vi "Set Wire Label.vi"(8 "error in (no error)":errorcluster, 9 "QD Combo Box Ref":refnum<vi>, 10 "Shift Not Pressed?":bool, 11 "Wire in":refnum<vi>) -> (0 "error out":errorcluster)   [LabVIEW 2017]
uses:
  <vilib>/Utility/miscctls.llb/LVPointTypeDef.ctl
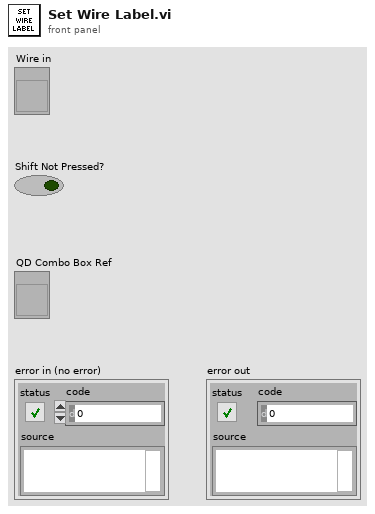
[diagram p1: front panel]
types:
  T1 = typedef "LVPointTypeDef.ctl" = cluster{"Horizontal":i16, "Vertical":i16}
  T2 = cluster{"Position":cluster{"h":i16, "v":i16}, "Flags":i32, "Type":enum32{"LooseEnd", "Endpoint", "Bend", "Junction"}, "Up Joint Index":i16, "Down Joint Index":i16, "Left Joint Index":i16, "Right Joint Index":i16}[]
  T3 = typedef "LVBoundsTypeDef.ctl" = cluster{"Width":u32, "Height":u32}
  T4 = cluster{"Position":cluster{"h":i16, "v":i16}, "Flags":i32, "Type":enum32{"LooseEnd", "Endpoint", "Bend", "Junction"}, "Up Joint Index":i16, "Down Joint Index":i16, "Left Joint Index":i16, "Right Joint Index":i16}
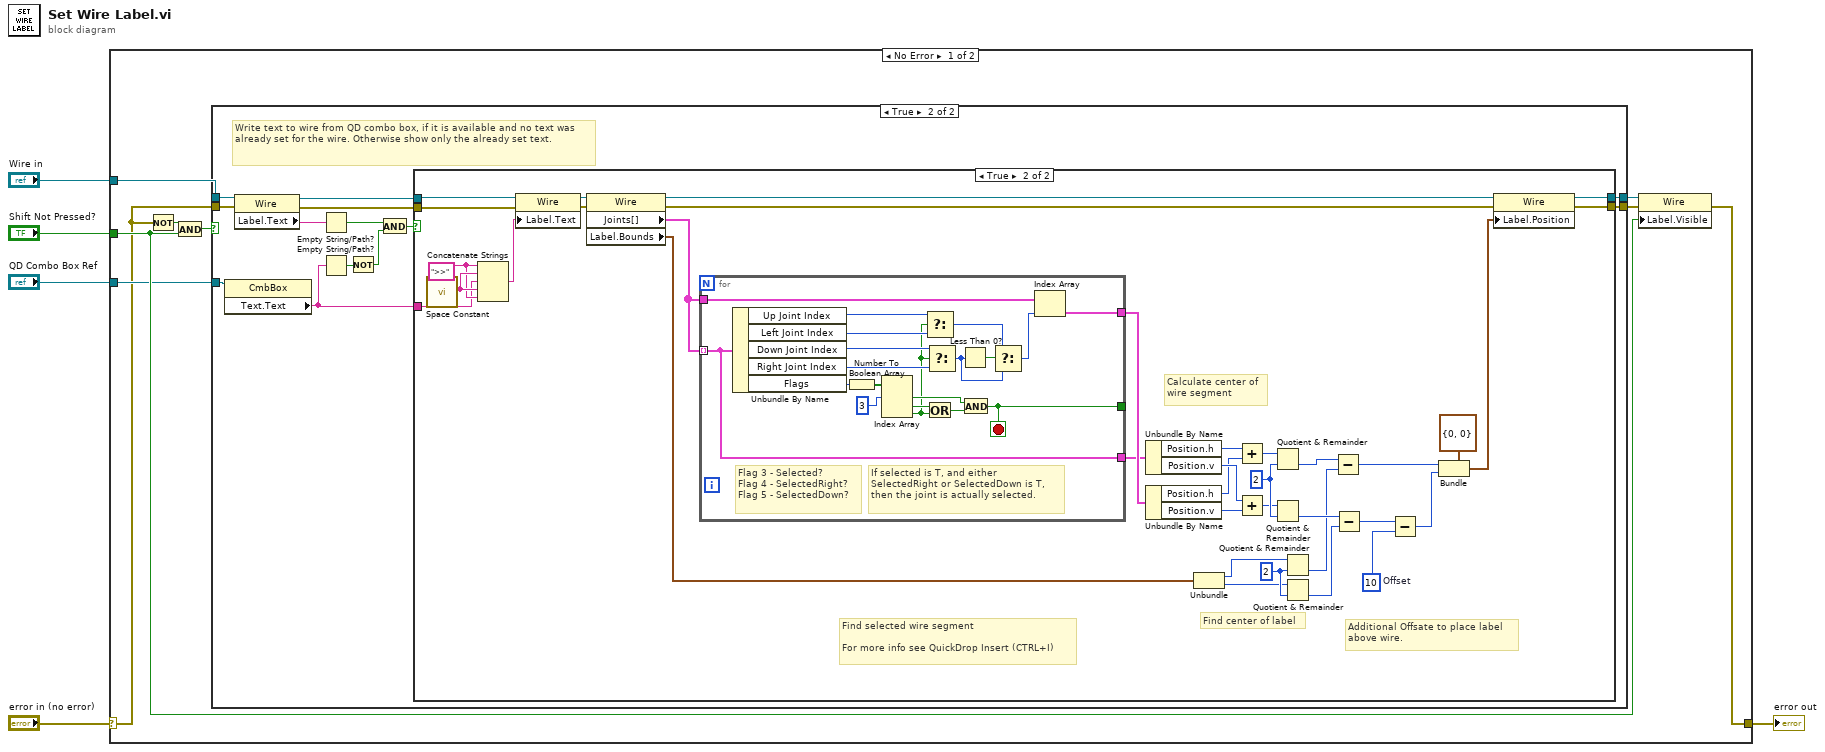
[diagram p0: block diagram]
diagram:
  n1 = case shown="No Error" "error in (no error)" {
    selector: "error in (no error)" -> [w12 w87]
    tunnel: [w6 w87] -> w5
    tunnel: "Shift Not Pressed?" -> [w14 _]
    tunnel: "QD Combo Box Ref" -> [w13 _]
    tunnel: "Wire in" -> [w7 _]
    frame No Error {
      n2 = Not(x=w12) -> (.not. x?=w11:bool)
      n3 = And(x=w11, y=w14) -> (x .and. y?=w10:bool)
      n4 = case shown="True" w10 {
        tunnel: w13 -> [_ w29]
        tunnel: w7 -> [w16 w26]
        tunnel: [w16 w28] -> w8
        tunnel: [w15 w27] -> w9
        tunnel: w12 -> [w15 w25]
        frame False {
        }
        frame True {
          # "Write text to wire from QD combo box, if it is available and no text was already set for the wire. Otherwise show only the already set text."
          n5 = property class="CmbBox"(reference=w29) -> ("Text.Text"=w21:string)  [unwired: 1 in, 2 out]
          n6 = property class="Wire"(reference=w26, error in=w25) -> (reference out=w23:refnum<vi>, error out=w24:errorcluster, "Label.Text"=w22:string)
          n7 = Empty String/Path?(string/path=w22) -> (empty?=w17:bool)
          n8 = Empty String/Path?(string/path=w21) -> (empty?=w20:bool)
          n9 = Not(x=w20) -> (.not. x?=w18:bool)
          n10 = And(x=w17, y=w18) -> (x .and. y?=w19:bool)
          n11 = case shown="True" w19 {
            tunnel: [w31 w48] -> w28
            tunnel: [w30 w47] -> w27
            tunnel: w24 -> [w30 w64]
            tunnel: w23 -> [w31 w63]
            tunnel: w21 -> [_ w62]
            frame False {
            }
            frame True {
              w36 = u32 10  # Offset
              w43 = i16 2 ("y")
              w56 = i16 2 ("y")
              w66 = ">>"
              # "Calculate center of\nwire segment"
              # "Find center of label"
              # "Additional Offsate to place label\nabove wire."
              # "Find selected wire segment\n\nFor more info see QuickDrop Insert (CTRL+I)"
              n12 = call <vilib>:"Space Constant.vi"() -> ("String"=w67:string)
              n13 = Concatenate Strings(w66, w67, w62, w67, w66) -> (w61:string)
              n14 = property class="Wire"(reference=w63, error in=w64, "Label.Text"=w61) -> (reference out=w65:refnum<vi>, error out=w59:errorcluster)
              n15 = property class="Wire"(reference=w65, error in=w59) -> (reference out=w60:refnum<vi>, error out=w46:errorcluster, "Joints[]"=w49:T2, "Label.Bounds"=w44:T3)
              n16 = for {
                tunnel: w49 -> [w80] mode=indexing
                tunnel: w49 -> [w79]
                tunnel: [w80] -> w51
                tunnel: [w78] -> w52
                tunnel: [w68] -> _
                stop <- w68 stop-if-true
                # "If selected is T, and either SelectedRight or SelectedDown is T, then the joint is actually selected."
                # "Flag 3 - Selected?\nFlag 4 - SelectedRight?\nFlag 5 - SelectedDown?"
                n17 = Unbundle By Name(w80) -> ("Up Joint Index"=w75:i16, "Left Joint Index"=w74:i16, "Down Joint Index"=w77:i16, "Right Joint Index"=w76:i16, "Flags"=w86:i32)
                n18 = Number To Boolean Array(number=w86) -> (Boolean array=w85:bool[])
                n19 = Index Array(array=w85, index #1=3 ("index")) -> (element #1=w81:bool, element #2=w82:bool, element #3=w73:bool)  [unwired: 2 in]
                n20 = Select(t=w75, s=w73, f=w74) -> (s? t:f=w70:i16)
                n21 = Or(x=w82, y=w73) -> (x .or. y?=w83:bool)
                n22 = Select(t=w77, s=w73, f=w76) -> (s? t:f=w69:i16)
                n23 = Less Than 0?(x=w69) -> (x < 0?=w71:bool)
                n24 = And(x=w81, y=w83) -> (x .and. y?=w68:bool)
                n25 = Select(t=w70, s=w71, f=w69) -> (s? t:f=w72:i16)
                n26 = Index Array(array=w79, index=w72) -> (element=w78:T4)
              }
              n27 = Unbundle By Name(w51) -> ("Position.h"=w35:i16, "Position.v"=w58:i16)
              n28 = Unbundle By Name(w52) -> ("Position.h"=w32:i16, "Position.v"=w33:i16)
              n29 = Unbundle(w44) -> ("Width"=w41:u32, "Height"=w42:u32)
              n30 = Add(x=w35, y=w32) -> (x+y=w53:i16)
              n31 = Add(x=w58, y=w33) -> (x+y=w55:i16)
              n32 = Quotient & Remainder(x=w53, y=w56) -> (floor(x/y)=w54:i16)  [unwired: 1 out]
              n33 = Quotient & Remainder(x=w55, y=w56) -> (floor(x/y)=w57:i16)  [unwired: 1 out]
              n34 = Quotient & Remainder(x=w41, y=w43) -> (floor(x/y)=w40:u32)  [unwired: 1 out]
              n35 = Quotient & Remainder(x=w42, y=w43) -> (floor(x/y)=w38:u32)  [unwired: 1 out]
              n36 = Subtract(x=w54, y=w40) -> (x-y=w34:u32)
              n37 = Subtract(x=w57, y=w38) -> (x-y=w39:u32)
              n38 = Subtract(x=w39, y=w36) -> (x-y=w37:u32)
              n39 = Bundle(cluster=T1 {"Horizontal"=0, "Vertical"=0} ("Insertion Point"), "Horizontal"=w34, "Vertical"=w37) -> (w45:T1)
              n40 = property class="Wire"(reference=w60, error in=w46, "Label.Position"=w45) -> (reference out=w48:refnum<vi>, error out=w47:errorcluster)
            }
          }
        }
      }
      n41 = property class="Wire"(reference=w8, error in=w9, "Label.Visible"=w14) -> (error out=w6:errorcluster)  [unwired: 1 out]
    }
    frame Error {
    }
  }
  "error out" <- w5
